vi "speedline vi.vi"(9 "customQueue":refnum<queue>, 11 "parentQueue":refnum<queue>) -> ()   [LabVIEW 2018]
uses:
  custom sub vis/speedlineData.ctl
panel:
  out "recircTemp":dbl(slide) caption="Recirculation Delta" scale=0.0..40.0
  out "Waveform Graph":dbl[][](graph)
  out "XY Graph":cluster{dbl[], dbl[]}[](graph)
  in  "createSpeedlines":bool
  in  "filter":bool
  in  "Speedlines":path
  out "dataTable":string[][](table)
  in  "channels":cluster{"massflow":i32, "PR":i32, "recirc":i32} caption="Channel Assignment" {"recirc" items=["time", "gearbox", "Recirculation temp", "volute exit surface", "oil tank", "Inlet average", "Outlet average", "V-cone", "inlet pressure", "outlet pressure", "Motor speed", "V-cone DP", "Motor power", "Accelerometer", "Hotwire", "oil pressure", "butterfly valve position", "ball valve position", "Legacy speed", "new Vcone", "V-Cone: CR001", "pressure ratio", "Ambient pressure", "Ambient temperature"]; "PR" items=["time", "gearbox", "Recirculation temp", "volute exit surface", "oil tank", "Inlet average", "Outlet average", "V-cone", "inlet pressure", "outlet pressure", "Motor speed", "V-cone DP", "Motor power", "Accelerometer", "Hotwire", "oil pressure", "butterfly valve position", "ball valve position", "Legacy speed", "new Vcone", "V-Cone: CR001", "pressure ratio", "Ambient pressure", "Ambient temperature"]; "massflow" items=["time", "gearbox", "Recirculation temp", "volute exit surface", "oil tank", "Inlet average", "Outlet average", "V-cone", "inlet pressure", "outlet pressure", "Motor speed", "V-cone DP", "Motor power", "Accelerometer", "Hotwire", "oil pressure", "butterfly valve position", "ball valve position", "Legacy speed", "new Vcone", "V-Cone: CR001", "pressure ratio", "Ambient pressure", "Ambient temperature"]}
  in  "really stop":bool
  in  "quit":bool
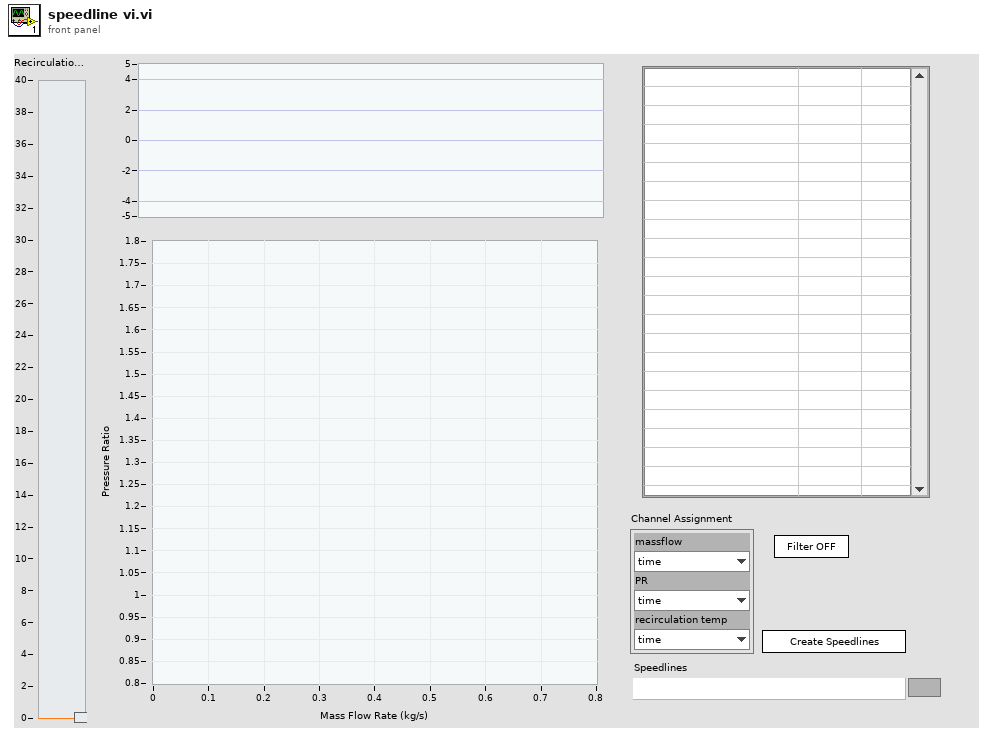
[diagram p1: front panel]
types:
  T1 = typedef "speedlineData.ctl" = cluster{"rigChannels":string[], "rigUnits":string[], "logging":bool, "chartRef":refnum<vi>, "dataTableRef":refnum<vi>, "channelCount":i32, "trendIndex":i32, "channels":cluster{"massflow":i32, "PR":i32, "recircTemp":i32}, "History":cluster{"speedlines":cluster{"mDot":dbl[], "pRatio":dbl[]}[], "liveTail":cluster{"mDot":dbl[], "pRatio":dbl[]}, "current":cluster{"mDot":dbl, "pRatio":dbl}, "insertPoint":i32, "tempHistory":dbl[][]}, "filter":bool, "filterLength":i32, "tableUpdate":i16, "limitValues":dbl[][]}
  T2 = cluster{"Pinlet":i32, "Poutlet":i32, "recircTemp":i32}
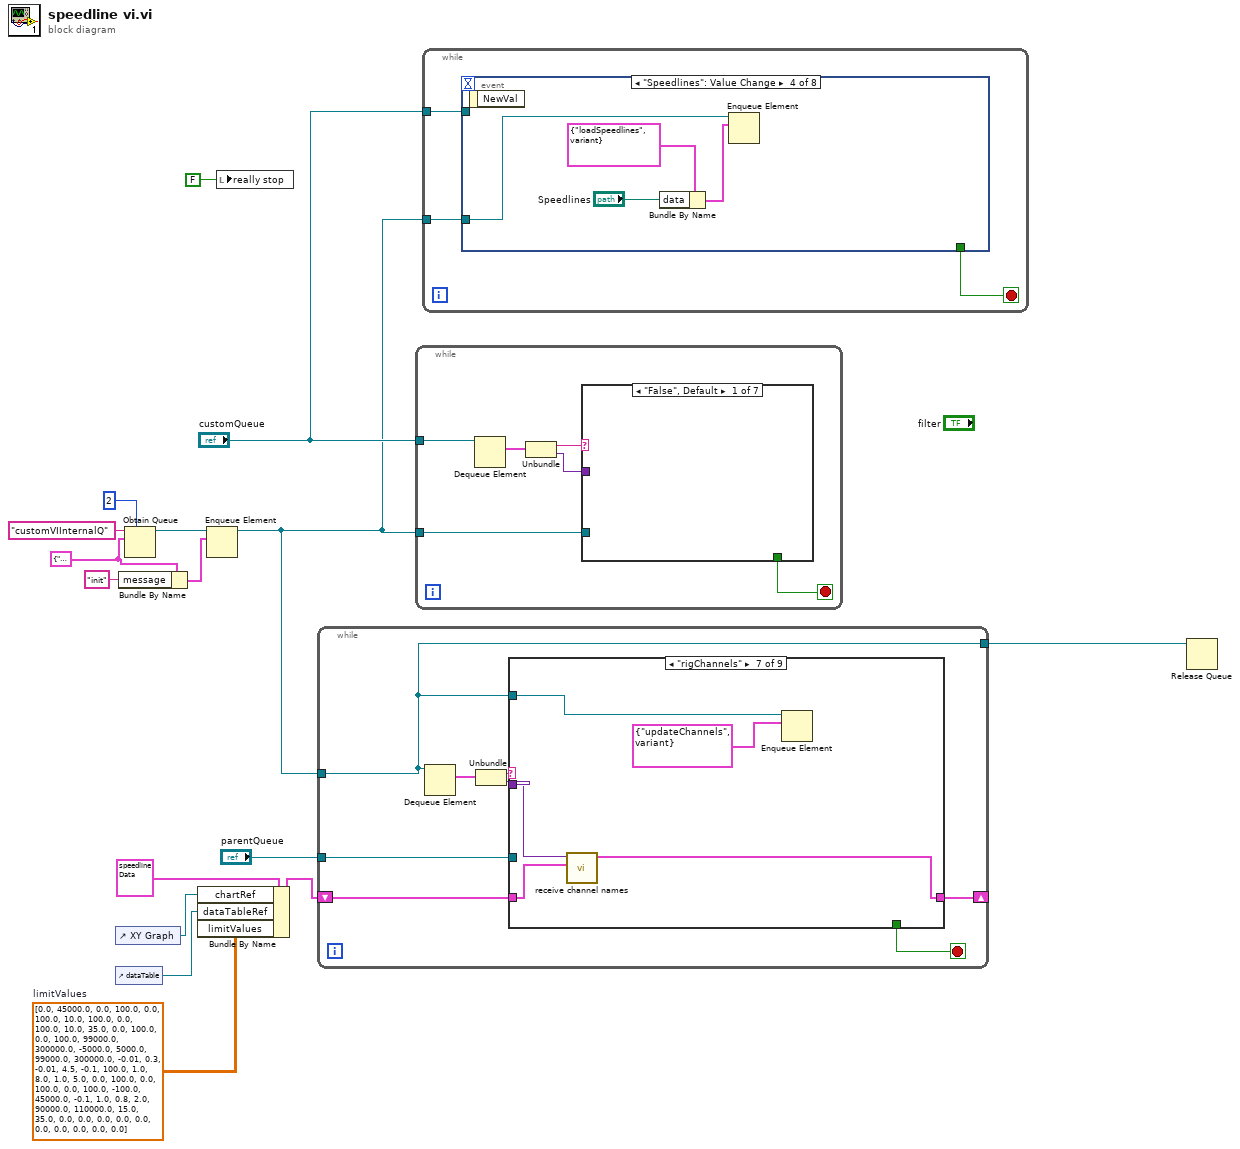
[diagram p0: block diagram]
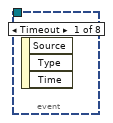
[diagram p2: hidden frame]
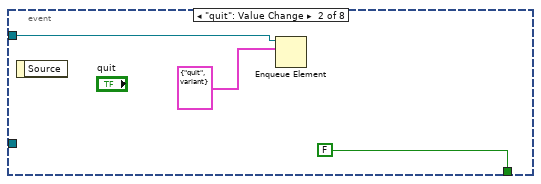
[diagram p3: hidden frame]
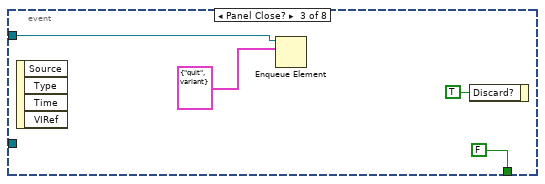
[diagram p4: hidden frame]
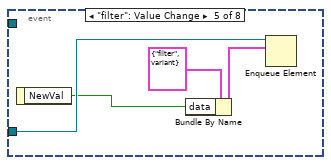
[diagram p5: hidden frame]
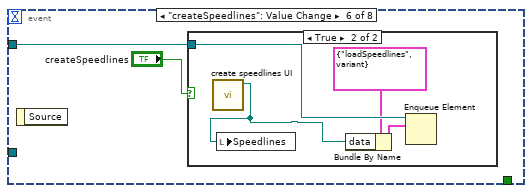
[diagram p6: hidden frame]
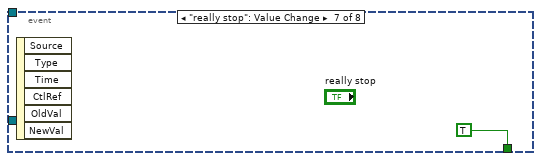
[diagram p8: hidden frame]
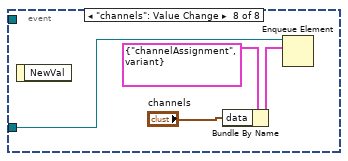
[diagram p9: hidden frame]
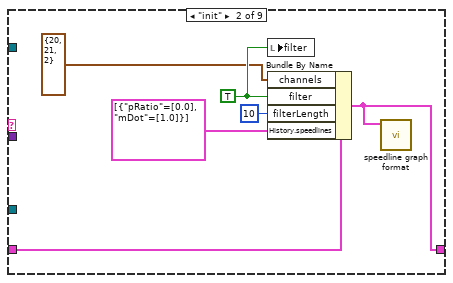
[diagram p11: hidden frame]
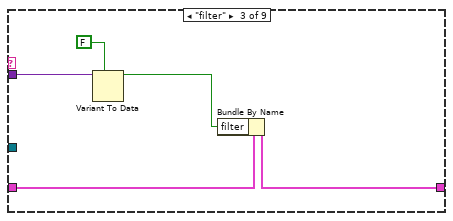
[diagram p12: hidden frame]
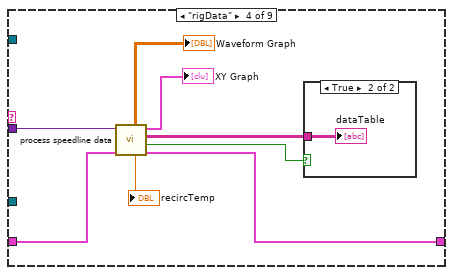
[diagram p13: hidden frame]
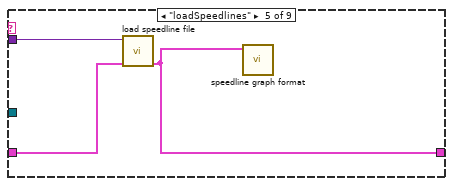
[diagram p15: hidden frame]
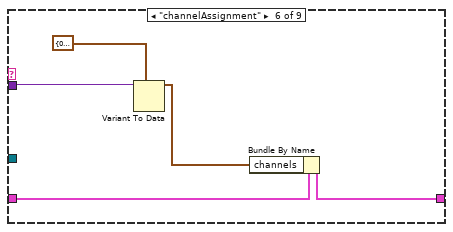
[diagram p16: hidden frame]
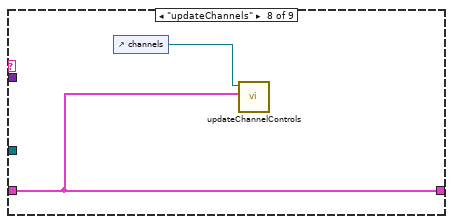
[diagram p17: hidden frame]
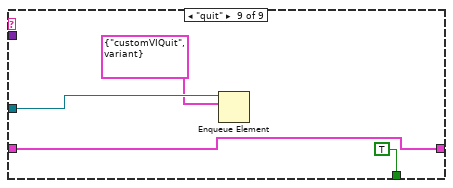
[diagram p18: hidden frame]
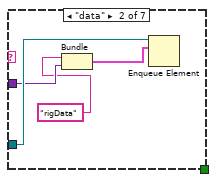
[diagram p19: hidden frame]
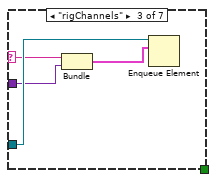
[diagram p20: hidden frame]
diagram:
  w1 = dbl[][] [[0.0, 45000.0], [0.0, 100.0], [0.0, 100.0], [10.0, 100.0], [0.0, 100.0], [10.0, 35.0], [0.0, 100.0], [0.0, 100.0], [99000.0, 300000.0], [-5000.0, 5000.0], [99000.0, 300000.0], [-0.01, 0.3], [-0.01, 4.5], [-0.1, 100.0], [1.0, 8.0], [1.0, 5.0], [0.0, 100.0], [0.0, 100.0], [0.0, 100.0], [-100.0, 45000.0], [-0.1, 1.0], [0.8, 2.0], [90000.0, 110000.0], [15.0, 35.0], [0.0, 0.0], [0.0, 0.0], [0.0, 0.0], [0.0, 0.0], [0.0, 0.0]]  # limitValues
  w8 = cluster{"message":string, "data":variant} {"message"="", "data"=variant} ("element")
  n1 = control-ref of="XY Graph"() -> (w3:refnum<vi>)
  n2 = control-ref of="dataTable"() -> (w2:refnum<vi>)
  n3 = Bundle By Name(cluster=w8, "message"="init") -> (w7:cluster{"message":string, "data":variant})
  n4 = Obtain Queue(max queue size (-1, unlimited)=2, name (unnamed)="customVIInternalQ", element data type=w8) -> (queue out=w14:refnum<queue>)  [unwired: 2 in, 2 out]
  n5 = Bundle By Name(cluster=T1 {"rigChannels"=[], "rigUnits"=[], "logging"=FALSE, "chartRef"=refnum, "dataTableRef"=refnum, "channelCount"=0, "trendIndex"=0, "channels"={"massflow"=0, "PR"=0, "recircTemp"=0}, "History"={"speedlines"=[], "liveTail"={"mDot"=[], "pRatio"=[]}, "current"={"mDot"=0.0, "pRatio"=0.0}, "insertPoint"=0, "tempHistory"=[]}, "filter"=FALSE, "filterLength"=0, "tableUpdate"=0, "limitValues"=[[0.0, 45000.0], [0.0, 100.0], [0.0, 100.0], [10.0, 100.0], [0.0, 100.0], [10.0, 35.0], [0.0, 100.0], [0.0, 100.0], [99000.0, 300000.0], [-5000.0, 5000.0], [99000.0, 300000.0], [-0.01, 0.3], [-0.01, 4.5], [-0.1, 100.0], [1.0, 8.0], [1.0, 5.0], [0.0, 100.0], [0.0, 100.0], [0.0, 100.0], [-100.0, 45000.0], [-0.1, 1.0], [0.8, 2.0], [90000.0, 110000.0], [15.0, 35.0], [0.0, 0.0], [0.0, 0.0], [0.0, 0.0], [0.0, 0.0]]}, "chartRef"=w3, "dataTableRef"=w2, "limitValues"=w1) -> (w4:T1)
  n6 = Enqueue Element(queue=w14, element=w7) -> (queue out=w9:refnum<queue>)  [unwired: 2 in, 2 out]
  n7 = local write "really stop"(FALSE) -> ()
  n8 = while {
    tunnel: w9 -> [w17]
    tunnel: "parentQueue" -> [w21]
    tunnel: [w17] -> w12
    shift-right: [w19] -> _
    shift-left: w4 -> [w18]
    stop <- w20 stop-if-true
    n9 = Dequeue Element(queue=w17) -> (element=w24:cluster{"message":string, "data":variant})  [unwired: 2 in, 3 out]
    n10 = Unbundle(w24) -> ("message"=w23:string, "data"=w22:variant)
    n11 = case shown="\"rigChannels\"" w23 {
      tunnel: w22 -> [_ _ w34 w44 w48 w51 w58 _ _]
      tunnel: w21 -> [_ _ _ _ _ _ _ _ w64]
      tunnel: [_ _ _ _ _ _ _ _ TRUE] -> w20
      tunnel: [w25 w28 w35 w42 w46 w52 w56 w60 w61] -> w19
      tunnel: w18 -> [w25 w31 w36 w43 w47 w53 w57 w60 w61]
      tunnel: w17 -> [_ _ _ _ _ _ w55 _ _]
      frame "", Default {
      }
      frame "init" {
        w27 = TRUE ("filter")
        n12 = local write "filter"(w27) -> ()
        n13 = Bundle By Name(cluster=w31, "channels"=T2 {"Pinlet"=20, "Poutlet"=21, "recircTemp"=2}, "filter"=w27, "filterLength"=10, "History.speedlines"=cluster{"pRatio":dbl[], "mDot":dbl[]}[] [{"pRatio"=[0.0], "mDot"=[1.0]}]) -> (w28:T1)
        n14 = call "speedline graph format.vi"("Cluster in"=w28) -> ()  [unwired: 11 in]
      }
      frame "filter" {
        n15 = Variant To Data(type=FALSE ("filter"), Variant=w34) -> (data=w32:bool)  [unwired: 1 in, 1 out]
        n16 = Bundle By Name(cluster=w36, "filter"=w32) -> (w35:T1)
      }
      frame "rigData" {
        n17 = call "process speedline data.vi"("Cluster in"=w43, "data"=w44) -> ("Cluster out"=w42:T1, "updateTable"=w38:bool, "dataTable"=w40:string[][], "plotData"=→"XY Graph":cluster{"pRatio":dbl[], "mDot":dbl[]}[], "Recirculation Delta"=→"recircTemp":dbl, "temp history"=→"Waveform Graph":dbl[][])  [unwired: 4 in]
        n18 = case shown="True" w38 {
          tunnel: w40 -> [_ w45]
          frame False {
          }
          frame True {
            "dataTable" <- w45
          }
        }
      }
      frame "loadSpeedlines" {
        n19 = call "load speedline file.vi"("Cluster in"=w47, "data"=w48) -> ("Cluster out"=w46:T1)  [unwired: 9 in]
        n20 = call "speedline graph format.vi"("Cluster in"=w46) -> ()  [unwired: 11 in]
      }
      frame "channelAssignment" {
        n21 = Variant To Data(type=T2 {"Pinlet"=0, "Poutlet"=0, "recircTemp"=0} ("channels"), Variant=w51) -> (data=w49:T2)  [unwired: 1 in, 1 out]
        n22 = Bundle By Name(cluster=w53, "channels"=w49) -> (w52:T1)
      }
      frame "rigChannels" {
        n23 = call "receive channel names.vi"("Cluster in"=w57, "data"=w58) -> ("Cluster out"=w56:T1)  [unwired: 9 in]
        n24 = Enqueue Element(queue=w55, element=cluster{"message":string, "data":variant} {"message"="updateChannels", "data"=variant}) -> ()  [unwired: 2 in, 3 out]
      }
      frame "updateChannels" {
        n25 = control-ref of="channels"() -> (w59:refnum<vi>)
        n26 = call "updateChannelControls.vi"("Cluster"=w60, "channels"=w59) -> ()  [unwired: 10 in]
      }
      frame "quit" {
        n27 = Enqueue Element(queue=w64, element=cluster{"message":string, "data":variant} {"message"="customVIQuit", "data"=variant}) -> ()  [unwired: 2 in, 3 out]
      }
    }
  }
  n28 = while {
    tunnel: "customQueue" -> [w70]
    tunnel: w9 -> [w67]
    stop <- w66 stop-if-true
    n29 = Dequeue Element(queue=w70) -> (element=w69:cluster{"message":string, "data":variant})  [unwired: 2 in, 3 out]
    n30 = Unbundle(w69) -> ("message"=w65:string, "data"=w68:variant)
    n31 = case shown="\"False\", Default" w65 {
      selector: w65 -> [_ _ w75 _ _ _ _]
      tunnel: w68 -> [_ w73 w77 w80 w82 w84 _]
      tunnel: w67 -> [_ w74 w78 _ _ _ w87]
      tunnel: [_ _ _ _ _ _ TRUE] -> w66
      frame "False", Default {
      }
      frame "data" {
        n32 = Bundle("rigData", "data"=w73) -> (w72:cluster{string, "data":variant})  [unwired: 1 in]
        n33 = Enqueue Element(queue=w74, element=w72) -> ()  [unwired: 2 in, 3 out]
      }
      frame "rigChannels" {
        n34 = Bundle(w75, "data"=w77) -> (w76:cluster{string, "data":variant})  [unwired: 1 in]
        n35 = Enqueue Element(queue=w78, element=w76) -> ()  [unwired: 2 in, 3 out]
      }
      frame "speedChange" {
        n36 = Variant To Data(type=0.0 ("y"), Variant=w80) -> ()  [unwired: 1 in, 2 out]
      }
      frame "butterflyChange" {
        n37 = Variant To Data(type=0.0 ("y"), Variant=w82) -> ()  [unwired: 1 in, 2 out]
      }
      frame "ballChange" {
        n38 = Variant To Data(type=0.0 ("y"), Variant=w84) -> ()  [unwired: 1 in, 2 out]
      }
      frame "quit" {
        n39 = property on="really stop" class="Bool (strict)"("Val(Sgnl)"=TRUE) -> ()  [unwired: 2 in, 2 out]
        n40 = Enqueue Element(queue=w87, element=cluster{"message":string, "data":variant} {"message"="quit", "data"=variant}) -> ()  [unwired: 2 in, 3 out]
      }
    }
  }
  n41 = while {
    tunnel: w9 -> [w91]
    tunnel: "customQueue" -> [w89]
    stop <- w90 stop-if-true
    n42 = event shown="[3] \"Speedlines\": Value Change" {
      selector: _ -> [_ _ _ _ _ _ _ _]
      dyn-events: _ -> [_ _ _ _ _ _ _ _]
      timeout: _ -> [_ _ _ _ _ _ _ _]
      tunnel: w91 -> [_ _ _ w100 w106 _ _ w117]
      tunnel: [_ FALSE FALSE _ _ _ TRUE _] -> w90
      tunnel: w89 -> [_ w92 w96 _ _ w108 _ _]
      event Timeout {
        n43 = event-data() -> ()  [unwired: 1 in, 3 out]
      }
      event "quit": Value Change {
        n44 = event-data() -> ()  [unwired: 1 in, 1 out]
        n45 = Enqueue Element(queue=w92, element=cluster{"message":string, "data":variant} {"message"="quit", "data"=variant}) -> ()  [unwired: 2 in, 3 out]
      }
      event Panel Close? {
        n46 = event-data() -> ()  [unwired: 1 in, 4 out]
        n47 = Enqueue Element(queue=w96, element=cluster{"message":string, "data":variant} {"message"="quit", "data"=variant}) -> ()  [unwired: 2 in, 3 out]
        n48 = event-data("Discard?"=TRUE) -> ()  [unwired: 1 in, 1 out]
      }
      event "Speedlines": Value Change {
        n49 = event-data() -> ()  [unwired: 1 in, 1 out]
        n50 = Bundle By Name(cluster=cluster{"message":string, "data":variant} {"message"="loadSpeedlines", "data"=variant} ("element"), "data"="Speedlines") -> (w101:cluster{"message":string, "data":variant})
        n51 = Enqueue Element(queue=w100, element=w101) -> ()  [unwired: 2 in, 3 out]
      }
      event "filter": Value Change {
        n52 = event-data() -> ("NewVal"=w103:bool)  [unwired: 1 in]
        n53 = Bundle By Name(cluster=cluster{"message":string, "data":variant} {"message"="filter", "data"=variant} ("element"), "data"=w103) -> (w104:cluster{"message":string, "data":variant})
        n54 = Enqueue Element(queue=w106, element=w104) -> ()  [unwired: 2 in, 3 out]
      }
      event "createSpeedlines": Value Change {
        n55 = event-data() -> ()  [unwired: 1 in, 1 out]
        n56 = case shown="True" "createSpeedlines" {
          tunnel: w108 -> [_ w112]
          frame False {
          }
          frame True {
            n57 = call "create speedlines UI.vi"() -> ("speedlineFile"=w109:path)  [unwired: 11 in]
            n58 = local write "Speedlines"(w109) -> ()
            n59 = Bundle By Name(cluster=cluster{"message":string, "data":variant} {"message"="loadSpeedlines", "data"=variant} ("element"), "data"=w109) -> (w110:cluster{"message":string, "data":variant})
            n60 = Enqueue Element(queue=w112, element=w110) -> ()  [unwired: 2 in, 3 out]
          }
        }
      }
      event "really stop": Value Change {
        n61 = event-data() -> ()  [unwired: 1 in, 6 out]
      }
      event "channels": Value Change {
        n62 = event-data() -> ()  [unwired: 1 in, 1 out]
        n63 = Bundle By Name(cluster=cluster{"message":string, "data":variant} {"message"="channelAssignment", "data"=variant} ("element"), "data"="channels") -> (w115:cluster{"message":string, "data":variant})
        n64 = Enqueue Element(queue=w117, element=w115) -> ()  [unwired: 2 in, 3 out]
      }
    }
  }
  n65 = Release Queue(queue=w12) -> ()  [unwired: 2 in, 3 out]
